vi "Area de un triangulo Henry Ati.vi"() -> ()   [LabVIEW 2020]
panel:
  in  "String":string
  out "Area del triangulo":dbl
  in  "Altura":dbl
  in  "Base":dbl
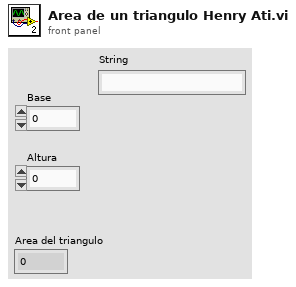
[diagram p1: front panel]
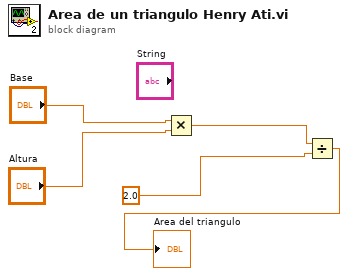
[diagram p0: block diagram]
diagram:
  n1 = Multiply(x="Base", y="Altura") -> (x*y=w5:dbl)
  n2 = Divide(x=w5, y=2.0) -> (x/y=→"Area del triangulo":dbl)
